vi "Exp_ICCD_SetOnChipAccumulations.vi"(8 "error in (no error)":errorcluster, 10 "On Chip Accumulations":i32, 11 "LightField Automation in":refnum<class "LightField Automation.lvclass">) -> (0 "error out":errorcluster, 3 "LightField Automation out":refnum<class "LightField Automation.lvclass">)   [LabVIEW 2019, in "LightField Automation.lvclass"]
uses:
  LightField Automation.lvclass
  C:/Program Files/Princeton Instruments/LightField/PrincetonInstruments.LightFieldAddInSupportServices.dll
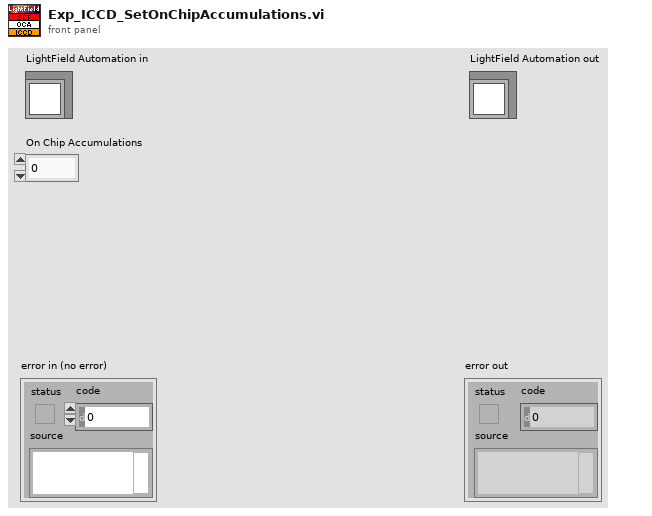
[diagram p1: front panel]
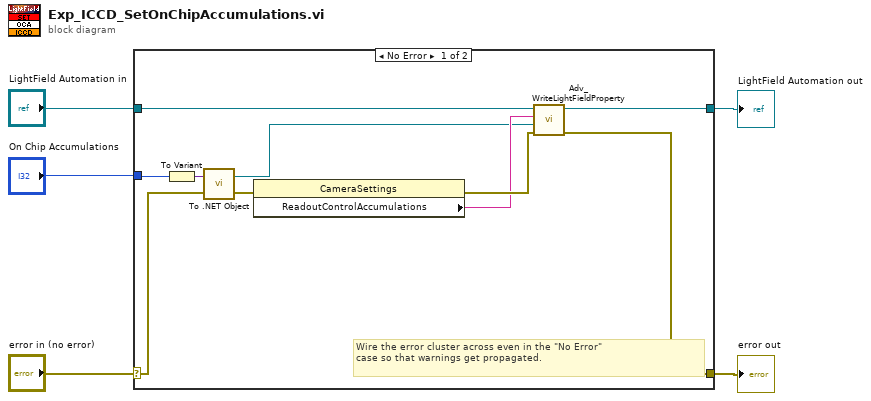
[diagram p0: block diagram]
diagram:
  n1 = case shown="No Error" "error in (no error)" {
    selector: "error in (no error)" -> [w6 w17]
    tunnel: [w7 w17] -> w4
    tunnel: [w11 w16] -> w2
    tunnel: "LightField Automation in" -> [w12 w16]
    tunnel: "On Chip Accumulations" -> [w15 _]
    frame No Error {
      # "Wire the error cluster across even in the \"No Error\"\ncase so that warnings get propagated."
      n2 = To Variant(anything=w15) -> (Variant=w14:variant)
      n3 = call <vilib>:"To .NET Object.vi"("error in (no error)"=w6, "anything"=w14) -> ("error out"=w13:errorcluster, ".NET object"=w8:refnum<k24>)
      n4 = property class="CameraSettings"(error in=w13) -> (error out=w10:errorcluster, "ReadoutControlAccumulations"=w9:string)  [unwired: 1 in, 1 out]
      n5 = call "Adv_WriteLightFieldProperty.vi"("error in (no error)"=w10, "value"=w8, "setting"=w9, "LightField Automation in"=w12) -> ("error out"=w7:errorcluster, "LightField Automation out"=w11:refnum<class "LightField Automation.lvclass">)  [unwired: 6 in]
    }
    frame Error {
    }
  }
  "error out" <- w4
  "LightField Automation out" <- w2
